vi "Pointer producer consumer Sun disk disable.vi"(0 "ADC0":dbl, 1 "ADC1":dbl, 2 "ADC2":dbl, 3 "ADC3":dbl) -> (6 "in - out":bool)   [LabVIEW 2014]
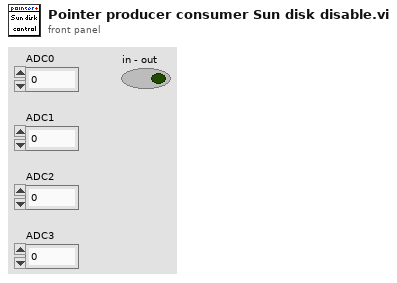
[diagram p1: front panel]
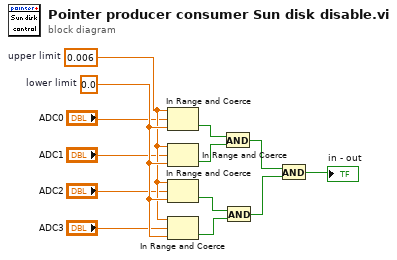
[diagram p0: block diagram]
diagram:
  w12 = 0.006  # upper limit
  w13 = 0.0  # lower limit
  n1 = In Range and Coerce(upper limit=w12, x="ADC0", lower limit=w13) -> (In Range?=w3:bool)  [unwired: 1 out]
  n2 = In Range and Coerce(upper limit=w12, x="ADC1", lower limit=w13) -> (In Range?=w4:bool)  [unwired: 1 out]
  n3 = In Range and Coerce(upper limit=w12, x="ADC2", lower limit=w13) -> (In Range?=w5:bool)  [unwired: 1 out]
  n4 = In Range and Coerce(upper limit=w12, x="ADC3", lower limit=w13) -> (In Range?=w6:bool)  [unwired: 1 out]
  n5 = And(x=w3, y=w4) -> (x .and. y?=w10:bool)
  n6 = And(x=w5, y=w6) -> (x .and. y?=w9:bool)
  n7 = And(x=w10, y=w9) -> (x .and. y?=→"in - out":bool)
